vi "IntakeReady.vi"() -> (3 "ReadyIndicator":bool)   [LabVIEW 2023]
doc: "The light will turn on when this Intake system is ready"
uses:
  IntakeGlobal.vi
  IntakeStates.ctl
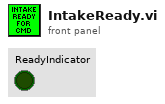
[diagram p1: front panel]
types:
  T1 = typedef "IntakeStates.ctl" = enum16{"Start", "WaitForCommand", "IntakeCoral", "IntakeAlgae", "WaitForCoral", "WaitForAlgae", "DepositCoral", "DepositAlgae", "DepositCoralTimer", "DepositAlgaeTimer"}
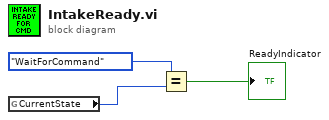
[diagram p0: block diagram]
diagram:
  n1 = global read "IntakeGlobal.vi" "CurrentState"() -> (w3:T1)
  n2 = Equal?(x=IntakeStates."WaitForCommand", y=w3) -> (x = y?=→"ReadyIndicator":bool)
